vi "Reports.vi"() -> ()   [LabVIEW 2018]
panel:
  in  "Down Button":bool
  in  "Up Button":bool
  out "Boolean 5":bool
  in  "Tank4":bool
  out "Boolean 4":bool
  in  "Tank2":bool
  out "Boolean 3":bool
  in  "Tank3":bool
  out "Boolean 2":bool
  in  "SideTank1":bool
  in  "Generate Detailed Document":bool
  in  "Generate Detailed Spreadsheet":bool
  in  "End Date 2":timestamp format="%<%I:%M %p\n%m/%d/%y>T"
  in  "Start Date 2":timestamp format="%<%I:%M %p\n%m/%d/%y>T"
  in  "End Date":timestamp format="%<%I:%M %p\n%m/%d/%y>T"
  in  "Start Date":timestamp format="%<%I:%M %p\n%m/%d/%y>T"
  in  "OK Button 2":bool
  in  "OK Button":bool
  out "Multicolumn Listbox":i32(listbox)=5
  in  "stop":bool
  # "Reports"
  # "Summary Report"
  # "Detailed Report"
  # "Enable Report for:"
  # "Fillings and Drains"
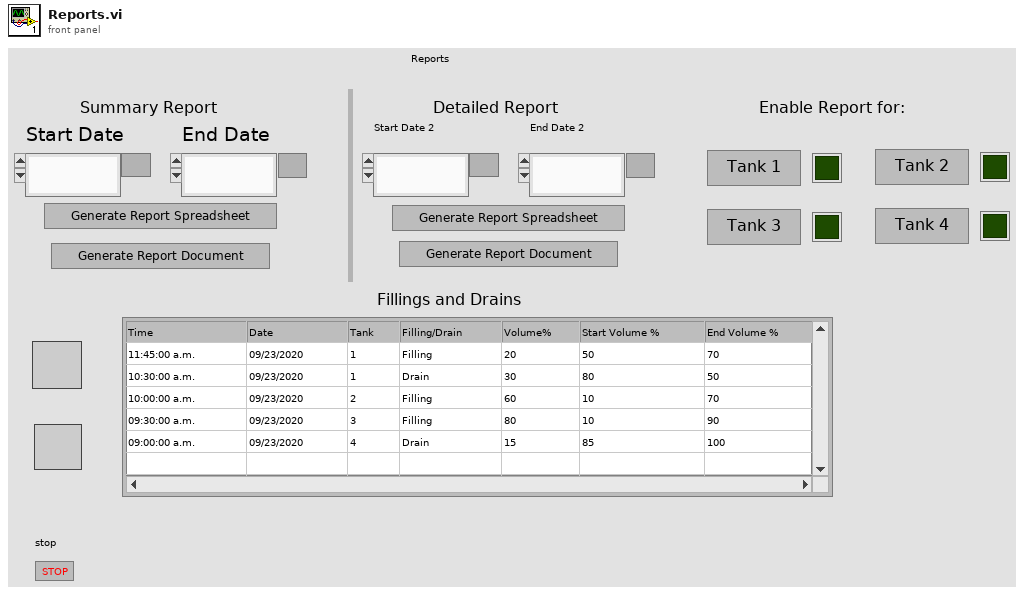
[diagram p1: front panel]
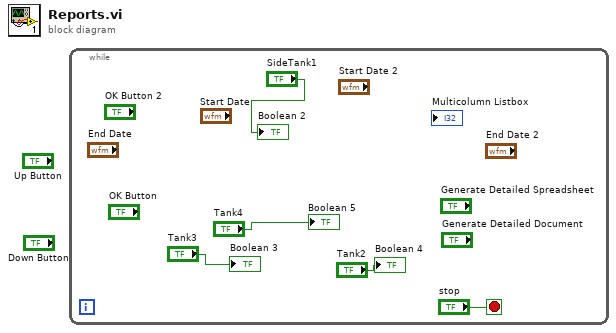
[diagram p0: block diagram]
diagram:
  n1 = while {
    stop <- "stop" stop-if-true
    "Boolean 2" <- "SideTank1"
    "Boolean 3" <- "Tank3"
    "Boolean 4" <- "Tank2"
    "Boolean 5" <- "Tank4"
  }
